vi "Generate merged movie.vi"(0 "Image colors":u32[](array[colorbox])=[16711680, 1048329], 2 "Display info in":T2(array[cluster]), 3 "Image info":T3(array[cluster])=[{"File name"=path "\\\\jg-i\\c-drive/LabView development/Glimpse/Test Data/Merge test/gelles00096full.tif", "TIFF stack?"=TRUE, "Frame # if stack?"=1}, {"File name"=path "\\\\jg-i\\c-drive/LabView development/Glimpse/Test Data/Merge test/gelles00097full.tif", "TIFF stack?"=TRUE, "Frame # if stack?"=1}], 4 "ROI":i32[](array[numeric])=[0, 0, 32767, 32767], 5 "Transform":u16(ring) items=["linear conformal", "affine", "projective"]) -> ()   [LabVIEW 2011]
doc: "Generates a merged pseudocolor AVI movie from two stacked tiffs."
uses:
  <vilib>/vision/Image Controls.llb/IMAQ Image.ctl
panel:
  in  "AVI compressors":i32(listbox)=11
  in  "Go!":bool
  in  "Frames Per Second":u32=30
  out "Current frame #":u32[](array[numeric])
  out "Max frames":i32[](array[numeric])
  in  "Write text overlay":bool=TRUE
  in  "stop":bool
  # "(Microsoft Video 1 works with Windows Media Player)"
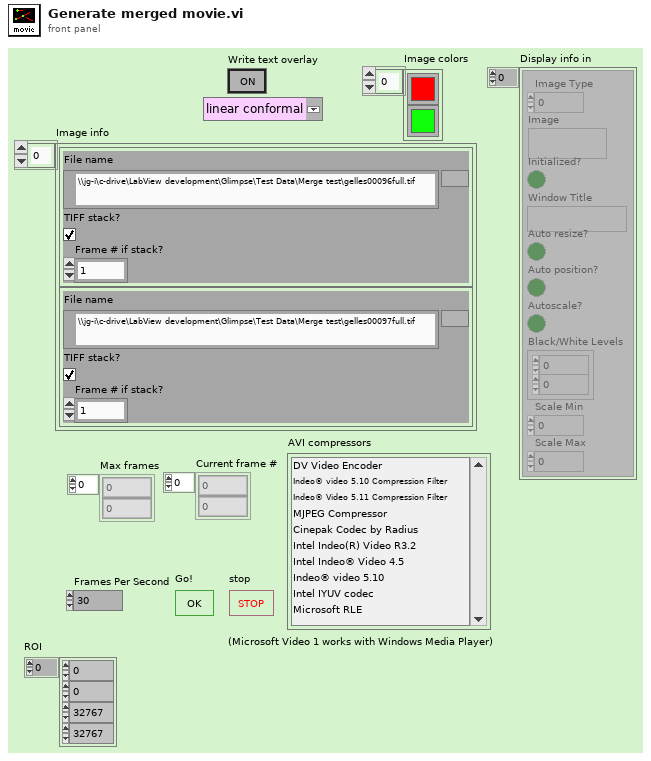
[diagram p1: front panel]
types:
  T1 = typedef "IMAQ Image.ctl" = refnum<image>
  T2 = cluster{"Image Type":u32, "Image":T1, "Initialized?":bool, "Window Title":string, "Auto resize?":bool, "Auto position?":bool, "Autoscale?":bool, "Black/White Levels":cluster{ext, ext}, "Scale Min":ext, "Scale Max":ext}[]
  T3 = cluster{"File name":path, "TIFF stack?":bool, "Frame # if stack?":u32}[]
  T4 = typedef "AviRefnum.ctl" = refnum<k1>
  T5 = typedef "Header file data.ctl" = cluster{"Frames Acquired":u32, "Region width":i32, "Region height":i32, "Element 0 of TTB":u32, "time of 1st frame, \nsec since 1/1/04":dbl, "TTB Array (ms)":u32[], "Offsets Array":T6, "Pixel depth":u32}
  T6 = typedef "Offset table.ctl" = cluster{"offset":T7, "file number":T8}[]
  T7 = typedef "Offset.ctl" = i32
  T8 = typedef "file number.ctl" = u8
  T9 = cluster{"File name":path, "TIFF stack?":bool, "Frame # if stack?":u32}
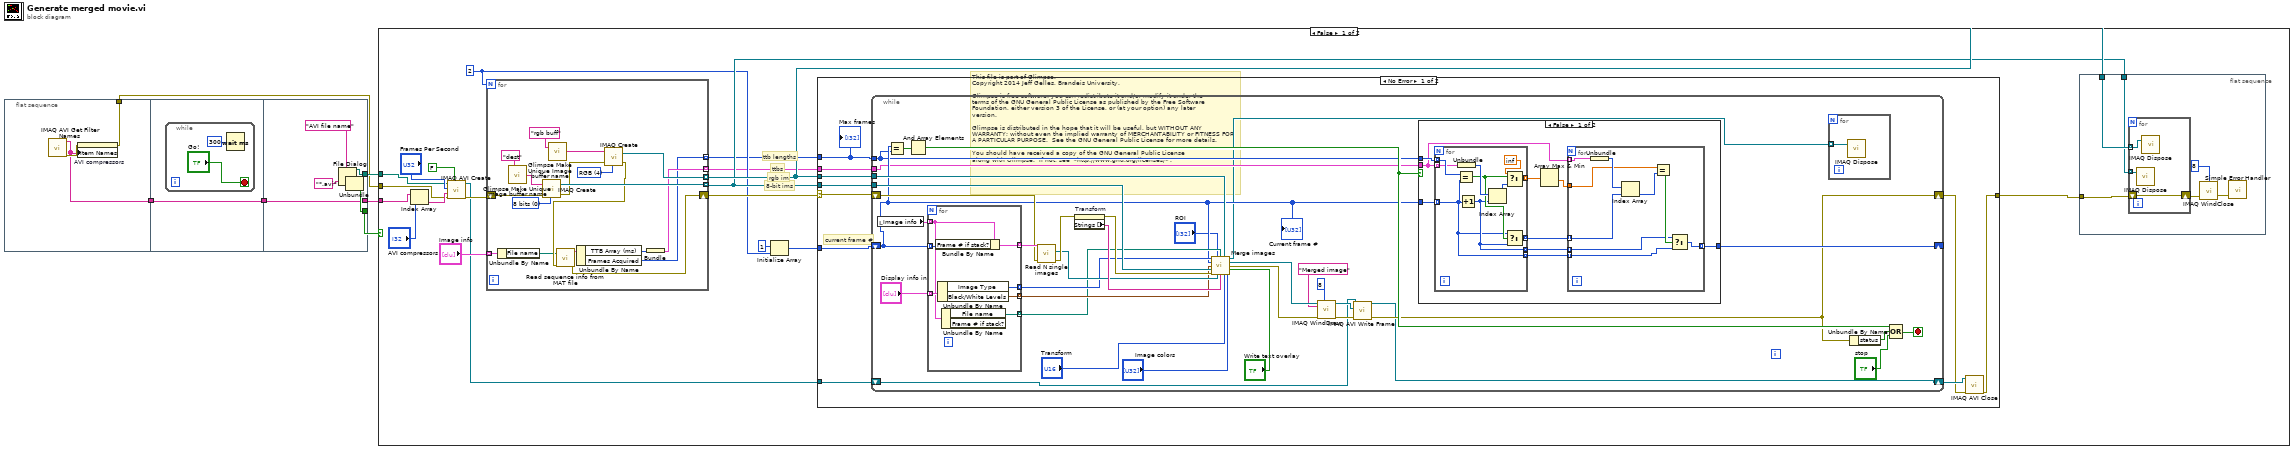
[diagram p0: block diagram]
diagram:
  # "This file is part of Glimpse. \nCopyright 2014 Jeff Gelles, Brandeis University.    \n\nGlimpse is free software: you can redistribute it and/or modify it under the \nterms of the GNU General Public License as published by the Free Software \nFoundation, either version 3 of the License, or (at your option) any later \nversion.\n\nGlimpse is distributed in the hope that it will be useful, but WITHOUT ANY \nWARRANTY; without even the implied warranty of MERCHANTABILITY or FITNESS FOR \nA PARTICULAR PURPOSE.  See the GNU General Public License for more details.\n\nYou should have received a copy of the GNU General Public License\nalong with Glimpse.  If not, see <http://www.gnu.org/licenses/>."
  n1 = flat-sequence {
    tunnel: [w8] -> w3
    tunnel: [w7] -> w1
    tunnel: w3 -> [w10]
    tunnel: [w10] -> w2
    tunnel: [w18] -> w6
    tunnel: [w17] -> w5
    tunnel: [w14] -> w4
    tunnel: w2 -> [w14]
    frame #0 {
      n2 = call "IMAQ AVI Get Filter Names"() -> ("error out"=w9:errorcluster, "Filter Names"=w8:string[])  [unwired: 1 in, 9 out]
      n3 = property on="AVI compressors" class="LstBox (strict)"(error in=w9, "Item Names"=w8) -> (error out=w7:errorcluster)  [unwired: 1 in, 1 out]
    }
    frame #1 {
      n4 = while {
        stop <- "Go!" stop-if-true
        n5 = Wait (ms)(milliseconds to wait=u32 300) -> ()  [unwired: 1 out]
      }
    }
    frame #2 {
      n6 = File Dialog(6:"*.avi" ("pattern"), 7:"AVI file name" ("prompt")) -> (0:w13:errorcluster, 1:w18:bool, 3:w17:path)  [unwired: 1 in, 5 out]
      n7 = Unbundle(w13) -> ()  [unwired: 3 out]
    }
  }
  n8 = case shown="False" w6 {
    tunnel: w5 -> [w24 _]
    tunnel: w4 -> [w22 _]
    tunnel: w1 -> [w21 _]
    frame False {
      w32 = 2
      # "ttb lengths"
      # "ttbs"
      # "rgb im"
      # "8-bit ims"
      n9 = Index Array(array=w22, index="AVI compressors") -> (element=w23:string)
      n10 = call "IMAQ AVI Create"("Has Data"=FALSE, "error in (no error)"=w21, "Compression Filter"=w23, "Frames Per Second"="Frames Per Second", "AVI Path"=w24) -> ("error out"=w25:errorcluster, "Avi Refnum"=w19:T4)  [unwired: 2 in, 3 out]
      n11 = for {
        N: w32 -> [_]
        shift-right: [w50] -> w33
        shift-left: w25 -> [w61]
        tunnel: [w60] -> w35 mode=indexing
        tunnel: [w58] -> w37 mode=indexing
        tunnel: "Image info" -> [w54] mode=indexing
        tunnel: [w49] -> w29 mode=indexing
        tunnel: [w47] -> w28 mode=indexing
        w59 = u32 4 items=["8 bits", "16 bits", "Float", "Complex", "RGB", "HSL"] ("Image Type")
        w62 = u32 0 items=["8 bits", "16 bits", "Float", "Complex", "RGB", "HSL"] ("Image Type")
        n12 = Unbundle By Name(w54) -> ("File name"=w52:path)
        n13 = call "Glimpse Make Unique Image buffer name.vi"("Buffer  base name"="dest") -> ("Image Name"=w64:string)  [unwired: 1 out]
        n14 = call "IMAQ Create"("Image Name"=w64, "Image Type"=w62, "error in (no error)"=w61) -> ("New Image"=w60:T1, "error out"=w55:errorcluster)  [unwired: 1 in, 1 out]
        n15 = call "Glimpse Make Unique Image buffer name.vi"("Buffer  base name"="rgb buff" ("Image Name")) -> ("Image Name"=w56:string)  [unwired: 1 out]
        n16 = call "IMAQ Create"("Image Name"=w56, "Image Type"=w59, "error in (no error)"=w55) -> ("New Image"=w58:T1, "error out"=w53:errorcluster)  [unwired: 1 in, 1 out]
        n17 = call "Read sequence info from MAT file.vi"("error in"=w53, "Movie file name"=w52) -> ("error out"=w50:errorcluster, "Header file data"=w51:T5)  [unwired: 8 out]
        n18 = Unbundle By Name(w51) -> ("TTB Array (ms)"=w48:u32[], "Frames Acquired"=w47:u32)
        n19 = Bundle("TTB Array (ms)"=w48) -> (w49:cluster{"TTB Array (ms)":u32[]})  [unwired: 1 in]
      }
      n20 = Initialize Array(u32 1 ("element"), w32) -> (w30:u32[])
      n21 = case shown="No Error" w33 {
        selector: w33 -> [w74 w148]
        tunnel: w35 -> [w73 _]
        tunnel: w37 -> [w72 _]
        tunnel: [w65 w148] -> w36
        tunnel: w30 -> [w71 _]
        tunnel: w29 -> [w70 _]
        tunnel: w28 -> [w69 _]
        tunnel: w19 -> [w68 _]
        frame No Error {
          # "current frame #"
          n22 = while {
            shift-right: [w80] -> w66
            shift-left: w74 -> [w99]
            tunnel: w73 -> [w110]
            tunnel: w72 -> [w109]
            shift-right: [w82] -> _
            shift-left: w71 -> [w85]
            tunnel: w70 -> [w83]
            tunnel: w69 -> [w84]
            shift-right: [w77] -> w67
            shift-left: w68 -> [w78]
            stop <- w87 stop-if-true
            n23 = local read "Image info"() -> (w101:T3)
            n24 = Equal?(x=w85, y=w84) -> (x = y?=w88:bool[])
            n25 = And Array Elements(Boolean array=w88) -> (logical AND=w86:bool)
            n26 = for {
              tunnel: w101 -> [w144] mode=indexing
              tunnel: w85 -> [w147] mode=indexing
              tunnel: [w146] -> w100 mode=indexing
              tunnel: "Display info in" -> [w145] mode=indexing
              tunnel: [w143] -> w95 mode=indexing
              tunnel: [w142] -> w94 mode=indexing
              tunnel: [w141] -> w93 mode=indexing
              n27 = Bundle By Name(cluster=w144, "Frame # if stack?"=w147) -> (w146:T9)
              n28 = Unbundle By Name(w145) -> ("Image Type"=w142:u32, "Black/White Levels"=w143:cluster{ext, ext})
              n29 = Unbundle By Name(w144) -> ("File name"=w141:path)  [unwired: 1 out]
            }
            n30 = call "Read N single images.vi"("error in"=w99, "Image info"=w100) -> ("error out"=w97:errorcluster, "Images out"=w96:T1[])  [unwired: 6 out]
            n31 = property on="Transform" class="Ring (strict)"(error in=w97) -> (error out=w102:errorcluster, "Strings []"=w103:string[])  [unwired: 1 in, 1 out]
            n32 = call "Merge images.vi"("Image types"=w94, "ROI"="ROI", "File paths"=w93, "RGB image buffers in"=w109, "Overlay frame numbers"=w85, "Black/white levels"=w95, "8 bit scratch images"=w110, "Write text overlay?"="Write text overlay", "error in"=w102, "N-bit images in"=w96, "Transform types"=w103, "Transform number?"="Transform", "Image colors"="Image colors") -> ("N-bit images out"=w76:T1[], "RGB Image out"=w105:T1, "error out"=w106:errorcluster)
            n33 = call "IMAQ WindDraw"("Window Number (0...15)"=8, "error in (no error)"=w106, "Title"="Merged image", "Image"=w105) -> ("error out"=w81:errorcluster, "Image Out (duplicate)"=w79:T1)  [unwired: 2 in, 4 out]
            n34 = call "IMAQ AVI Write Frame"("error in (no error)"=w81, "Image"=w79, "Avi Refnum"=w78) -> ("error out"=w80:errorcluster, "Avi Refnum (duplicate)"=w77:T4)  [unwired: 1 in, 6 out]
            n35 = case shown="False" w86 {
              tunnel: w85 -> [w120 w140]
              tunnel: w84 -> [w119 _]
              tunnel: w83 -> [w117 _]
              tunnel: [w113 w140] -> w82
              frame False {
                n36 = for {
                  tunnel: w120 -> [w130] mode=indexing
                  tunnel: w119 -> [w139] mode=indexing
                  tunnel: w117 -> [w137] mode=indexing
                  tunnel: [w134] -> w118 mode=indexing
                  tunnel: [w132] -> w116 mode=indexing
                  tunnel: [w131] -> w115 mode=indexing
                  tunnel: [w130] -> w114 mode=indexing
                  n37 = Equal?(x=w139, y=w130) -> (x = y?=w133:bool)
                  n38 = Unbundle(w137) -> ("TTB Array (ms)"=w135:u32[])
                  n39 = Increment(x=w130) -> (x+1=w131:u32)
                  n40 = Index Array(array=w135, index=w131) -> (element=w136:u32)
                  n41 = Select(t=inf, s=w133, f=w136) -> (s? t:f=w134:dbl)
                  n42 = Select(t=w130, s=w133, f=w131) -> (s? t:f=w132:u32)
                }
                n43 = Array Max & Min(array=w118) -> (min value=w112:dbl)  [unwired: 3 out]
                n44 = for {
                  tunnel: w112 -> [w124]
                  tunnel: w117 -> [w127] mode=indexing
                  tunnel: w116 -> [w126] mode=indexing
                  tunnel: w115 -> [w123] mode=indexing
                  tunnel: w114 -> [w122] mode=indexing
                  tunnel: [w121] -> w113 mode=indexing
                  n45 = Unbundle(w127) -> ("TTB Array (ms)"=w129:u32[])
                  n46 = Index Array(array=w129, index=w126) -> (element=w125:u32)
                  n47 = Equal?(x=w124, y=w125) -> (x = y?=w128:bool)
                  n48 = Select(t=w123, s=w128, f=w122) -> (s? t:f=w121:u32)
                }
              }
              frame True {
              }
            }
            n49 = for {
              tunnel: w76 -> [w111] mode=indexing
              n50 = call "IMAQ Dispose"("Image"=w111) -> ()  [unwired: 2 in, 4 out]
            }
            n51 = Unbundle By Name(w80) -> ("status"=w89:bool)
            n52 = Compound Arithmetic op=OR(w86, w89, "stop") -> (w87:bool)
            "Current frame #" <- w85
          }
          n53 = call "IMAQ AVI Close"("error in (no error)"=w66, "Avi Refnum"=w67) -> ("error out"=w65:errorcluster)  [unwired: 9 out]
          "Max frames" <- w69
        }
        frame Error {
        }
      }
      n54 = flat-sequence {
        tunnel: w37 -> [w43]
        tunnel: w36 -> [w42]
        tunnel: w35 -> [w41]
        frame #0 {
          n55 = for {
            tunnel: w43 -> [w45] mode=indexing
            shift-right: [w46] -> w40
            shift-left: w42 -> [w46]
            tunnel: w41 -> [w44] mode=indexing
            n56 = call "IMAQ Dispose"("Image"=w44) -> ()  [unwired: 2 in, 4 out]
            n57 = call "IMAQ Dispose"("Image"=w45) -> ()  [unwired: 2 in, 4 out]
          }
          n58 = call "IMAQ WindClose"("Window Number (0...15)"=8, "error in (no error)"=w40) -> ("error out"=w38:errorcluster)  [unwired: 1 in, 3 out]
          n59 = call <vilib>:"Simple Error Handler.vi"("error in (no error)"=w38) -> ()  [unwired: 1 in, 8 out]
        }
      }
    }
    frame True {
    }
  }
